vi "CreateNumArray.vi"(1 "Offset":i32, 2 "Randomize?":bool, 3 "Steps":i32) -> (0 "Result":i32[](array[numeric]))   [LabVIEW 2013]
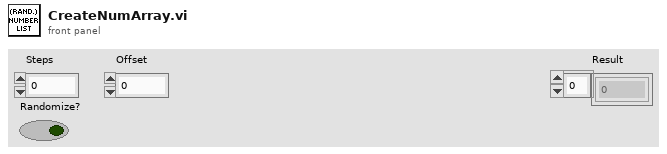
[diagram p1: front panel]
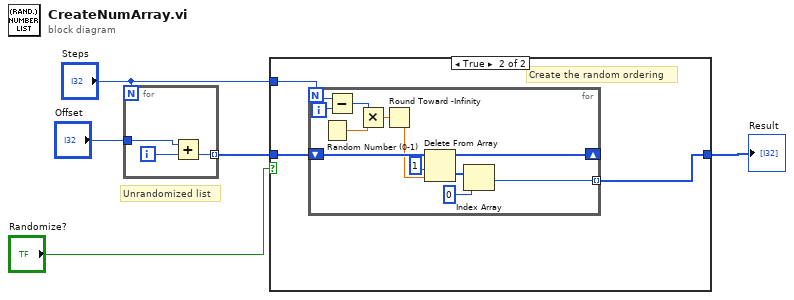
[diagram p0: block diagram]
diagram:
  # "Unrandomized list"
  n1 = for {
    N: "Steps" -> [_]
    tunnel: [w7] -> w4 mode=indexing
    tunnel: "Offset" -> [w6]
    i -> [w8]
    n2 = Add(x=w6, y=w8) -> (x+y=w7:i32)
  }
  n3 = case shown="True" "Randomize?" {
    tunnel: "Steps" -> [_ w12]
    tunnel: w4 -> [w9 w11]
    tunnel: [w9 w10] -> w2
    frame False {
    }
    frame True {
      # "Create the random ordering"
      n4 = for {
        N: w12 -> [w23]
        shift-right: [w18] -> _
        shift-left: w11 -> [w19]
        tunnel: [w13] -> w10 mode=indexing
        i -> [w24]
        n5 = Random Number (0-1)() -> (number: 0 to 1=w22:dbl)
        n6 = Subtract(x=w23, y=w24) -> (x-y=w21:i32)
        n7 = Multiply(x=w21, y=w22) -> (x*y=w20:dbl)
        n8 = Round Toward -Infinity(1:w20) -> (0:w16:dbl)
        n9 = Delete From Array(array=w19, length=1, index=w16) -> (deleted portion=w15:i32[], array with subset deleted=w18:i32[])
        n10 = Index Array(array=w15, index=0) -> (element=w13:i32)
      }
    }
  }
  "Result" <- w2
